vi "readRawFile.vi"() -> ()   [LabVIEW 2017]
panel:
  out "Error out":errorcluster
  in  "Raw File Path":path=path "F:/BonTechWrapperLibrary/BonTechWrapperLibrary/x64/Release/test.raw"
  in  "Length":i32=256
  in  "Frame Header":bool
  out "Image":T1(plugin-control)
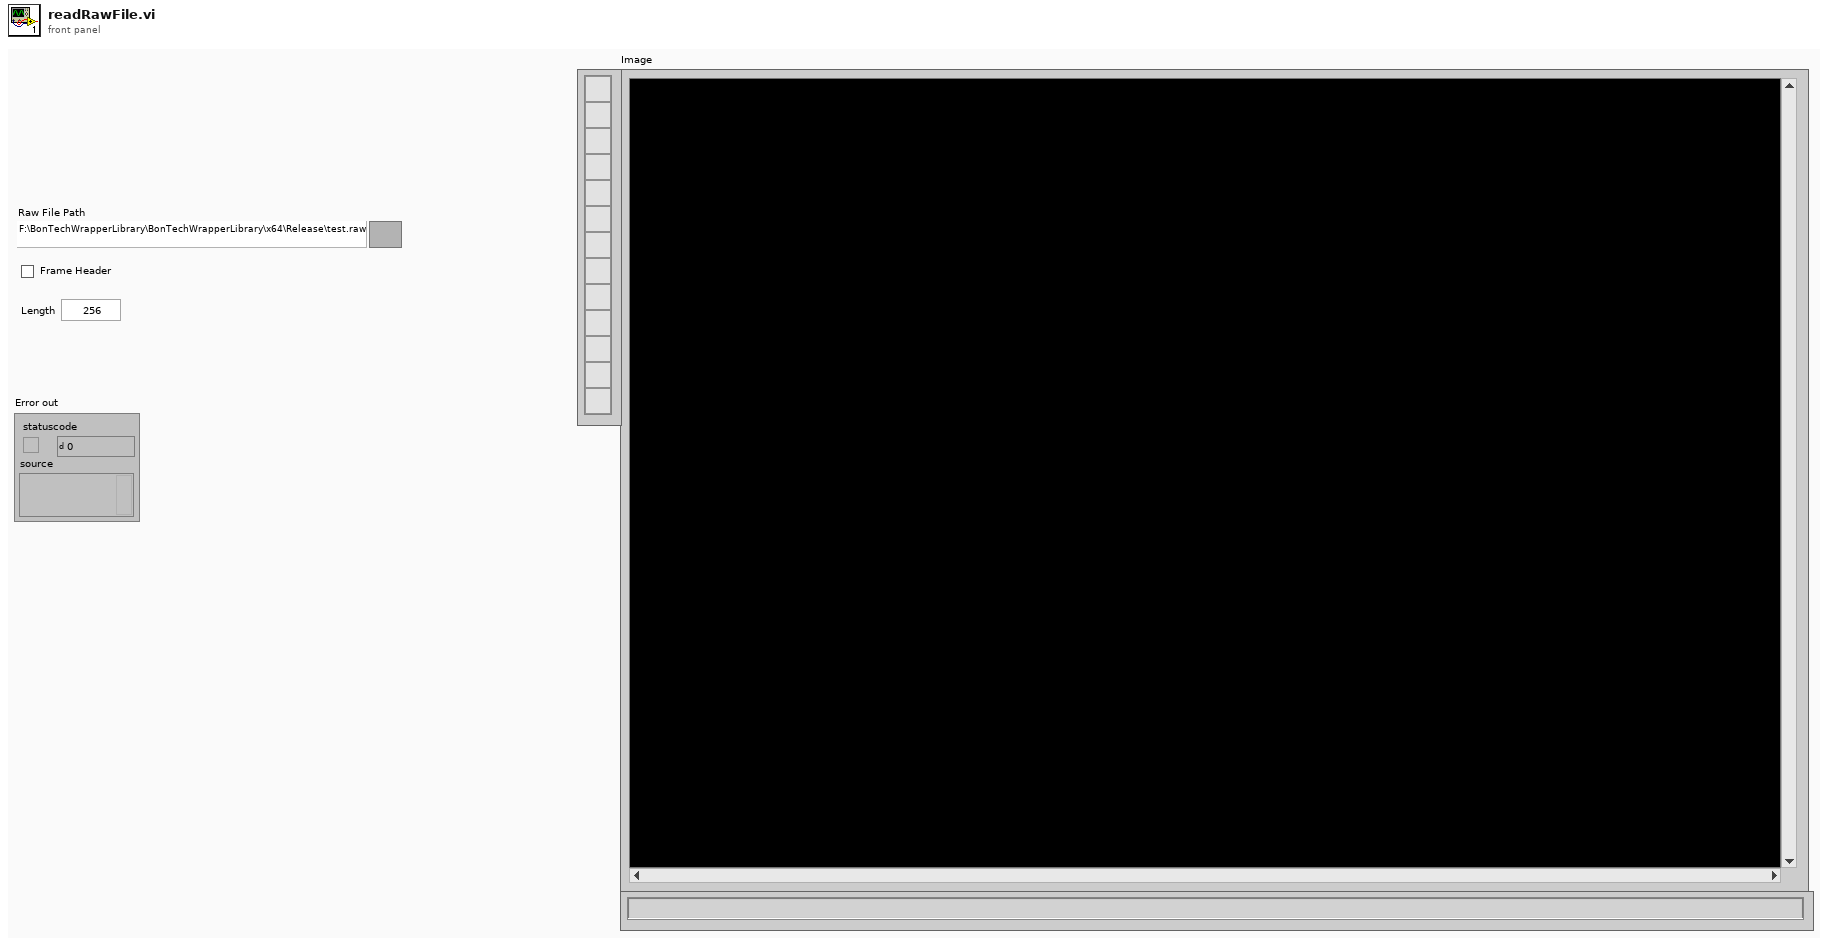
[diagram p1: front panel]
types:
  T1 = typedef "IMAQ Image.ctl" = refnum<image>
  T2 = typedef "Image Type" = u32
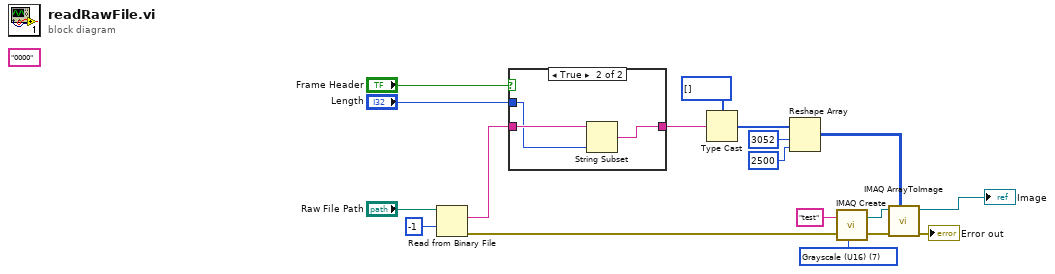
[diagram p0: block diagram]
diagram:
  w14 = T2 7 items=["Grayscale (U8)", "Grayscale (I16)", "Grayscale (SGL)", "Complex (CSG)", "RGB (U32)", "HSL (U32)", "RGB (U64)", "Grayscale (U16)"] ("Image Type")
  (unwired) "0000"
  n1 = Read from Binary File(10:-1 ("count (1)"), 11:"Raw File Path") -> (0:w2:errorcluster, 2:w5:string)  [unwired: 4 in, 2 out]
  n2 = case shown="True" "Frame Header" {
    tunnel: w5 -> [w19 w22]
    tunnel: "Length" -> [_ w21]
    tunnel: [w19 w20] -> w3
    frame False {
    }
    frame True {
      n3 = String Subset(string=w22, length (rest)=w21) -> (substring=w20:string)  [unwired: 1 in]
    }
  }
  n4 = Type Cast(type=u16[] [], x=w3) -> (*(type *) &x=w11:u16[])
  n5 = Reshape Array(w11, 3052 ("dimension size"), 2500 ("dimension size")) -> (w8:u16[][])
  n6 = call "IMAQ Create"("Image Name"="test", "Image Type"=w14, "error in (no error)"=w2) -> ("New Image"=w13:T1, "error out"=w7:errorcluster)  [unwired: 2 in]
  n7 = call "IMAQ ArrayToImage"("Image Pixels (U16)"=w8, "error in (no error)"=w7, "Image"=w13) -> ("error out"=→"Error out":errorcluster, "Image Out"=→"Image":T1)  [unwired: 7 in]
